vi "ryangosling.vi"(11 "CHASSIS":T6 {"vOmega" format="%10.3f"; "vY" format="%10.3f"; "vX" format="%10.3f"}) -> (1 "out WheelStates":T1[](array[typedef]) {"Angle"."SIN" format="%13.4f"; "Angle"."COS" format="%13.4f"; "Angle"."VALUE" format="%13.4f"}, 3 "out SWERVE_DRIVE_KINEMATICS":T3 {"SavedModuleStates"."Angle"."SIN" format="%13.4f"; "SavedModuleStates"."Angle"."COS" format="%13.4f"; "SavedModuleStates"."Angle"."VALUE" format="%13.4f"; "PrevCoR"."Y" format="%14.3f"; "PrevCoR"."X" format="%14.3f"; "Modules"."Y" format="%14.3f"; "Modules"."X" format="%14.3f"})   [LabVIEW 2023]
uses:
  <vilib>/Rock Robotics/WPI/ThirdParty/JAS_Junk/TrajLib/TypeDef/CHASSIS_SPEEDS.ctl
  <vilib>/Rock Robotics/WPI/ThirdParty/JAS_Junk/TrajLib/TypeDef/SWERVE_DRIVE_KINEMATICS.ctl
  <vilib>/Analysis/Matrix/Datatypes/RealMatrix.ctl
  <vilib>/Rock Robotics/WPI/ThirdParty/JAS_Junk/TrajLib/TypeDef/TRANSLATION2D.ctl
  <vilib>/Rock Robotics/WPI/ThirdParty/JAS_Junk/TrajLib/TypeDef/SWERVE_DRIVE_MODULE_STATE.ctl
  <vilib>/Rock Robotics/WPI/ThirdParty/JAS_Junk/TrajLib/TypeDef/ROTATION2D.ctl
  <vilib>/Rock Robotics/WPI/ThirdParty/JAS_Junk/TrajLib/Rotation2d_Minus.vi
  <vilib>/Rock Robotics/WPI/ThirdParty/JAS_Junk/TrajLib/Rotation2d_GetRadians.vi
  <vilib>/Rock Robotics/WPI/ThirdParty/JAS_Junk/TrajLib/SwerveModuleState_New.vi
  <vilib>/Rock Robotics/WPI/ThirdParty/JAS_Junk/TrajLib/Rotation2d_RotateBy.vi
  <vilib>/Rock Robotics/WPI/ThirdParty/JAS_Junk/TrajLib/Rotation2d_UnaryMinus.vi
  <vilib>/Rock Robotics/WPI/ThirdParty/JAS_Junk/TrajLib/Rotation2d_CreateXY.vi
  <vilib>/Rock Robotics/WPI/ThirdParty/JAS_Junk/TrajLib/Util_CalcDist.vi
  <vilib>/Rock Robotics/WPI/ThirdParty/JAS_Junk/TrajLib/Trajectory_Library.lvlib
  <vilib>/Rock Robotics/WPI/ThirdParty/REV Robotics/REVLib/Typedef/Spark MAX Control Type.ctl
  <vilib>/Analysis/Matrix/NI_Matrix.lvlib
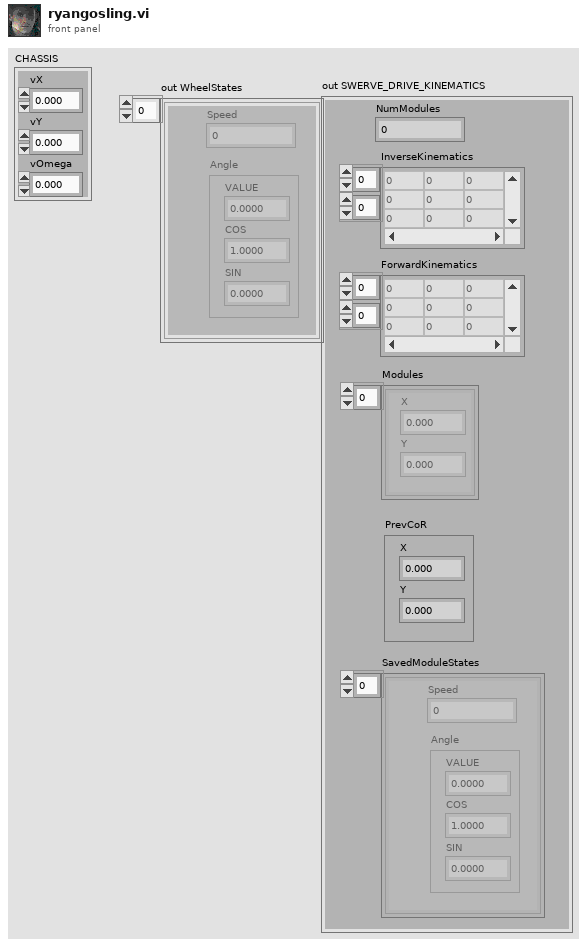
[diagram p1: front panel]
types:
  T1 = typedef "Trajectory_Library.lvlib/SWERVE_DRIVE_MODULE_STATE.ctl" = cluster{"Speed":dbl, "Angle":T2}
  T2 = typedef "Trajectory_Library.lvlib/ROTATION2D.ctl" = cluster{"VALUE":dbl, "COS":dbl, "SIN":dbl}
  T3 = typedef "Trajectory_Library.lvlib/SWERVE_DRIVE_KINEMATICS.ctl" = cluster{"NumModules":i32, "InverseKinematics":T4, "ForwardKinematics":T4, "Modules":T5[], "PrevCoR":T5, "SavedModuleStates":T1[]}
  T4 = typedef "NI_Matrix.lvlib/RealMatrix.ctl" = dbl[][]
  T5 = typedef "Trajectory_Library.lvlib/TRANSLATION2D.ctl" = cluster{"X":dbl, "Y":dbl}
  T6 = typedef "Trajectory_Library.lvlib/CHASSIS_SPEEDS.ctl" = cluster{"vX":dbl, "vY":dbl, "vOmega":dbl}
  T7 = typedef "WPI_MotorControlDeviceRef.ctl" = cluster{"DeviceStatus":errorcluster, "Type":T8, "PWM":cluster{"PWM Channel":T9, "DeadBand":T10}, "CAN":cluster{"Device Number":u8, "SetOutput VI Ref":variant, "GetOutput VI Ref":variant, "Enable VI Ref":variant, "Disable VI Ref":variant, "Data":variant}, "Invert":bool, "DIO PWM":cluster{"PWM \"Enable\" Channel":T9, "DIOChannel":T11, "PWM Rate":dbl}}
  T8 = typedef "WPI_MotorControlType.ctl" = enum16{"PWM", "CAN", "DIO PWM"}
  T9 = typedef "FPGA_DIOPWMChannel.ctl" = enum8{"PWM 0", "PWM 1", "PWM 2", "PWM 3", "PWM 4", "PWM 5", "PWM 6", "PWM 7", "PWM 8", "PWM 9", "PWM MXP 0", "PWM MXP 1", "PWM MXP 2", "PWM MXP 3", "PWM MXP 4", "PWM MXP 5", "PWM MXP 6", "PWM MXP 7", "PWM MXP 8", "PWM MXP 9", "Invalid"}
  T10 = typedef "WPI_PWMDeadband.ctl" = cluster{"Name":string, "maxPositivePwm":i32, "minPositivePwm":i32, "centerPwm":i32, "maxNegativePwm":i32, "minNegativePwm":i32, "angularRange":u16}
  T11 = typedef "FPGA_DIOChannel.ctl" = enum8{"DIO 0", "DIO 1", "DIO 2", "DIO 3", "DIO 4", "DIO 5", "DIO 6", "DIO 7", "DIO 8", "DIO 9", "DIO MXP 0", "DIO MXP 1", "DIO MXP 2", "DIO MXP 3", "DIO MXP 4", "DIO MXP 5", "DIO MXP 6", "DIO MXP 7", "DIO MXP 8", "DIO MXP 9", "DIO MXP 10", "DIO MXP 11", "DIO MXP 12", "DIO MXP 13", "DIO MXP 14", "DIO MXP 15", "SPI Port CS1", "SPI Port CS2", "SPI Port CS3", "SPI Port MISO", "SPI Port MOSI", "Invalid"}
  T12 = typedef "Spark MAX Control Type.ctl" = enum16{"Percent VBus", "Voltage", "Velocity", "Position", "Smart Motion", "Current", "Smart Velocity"}
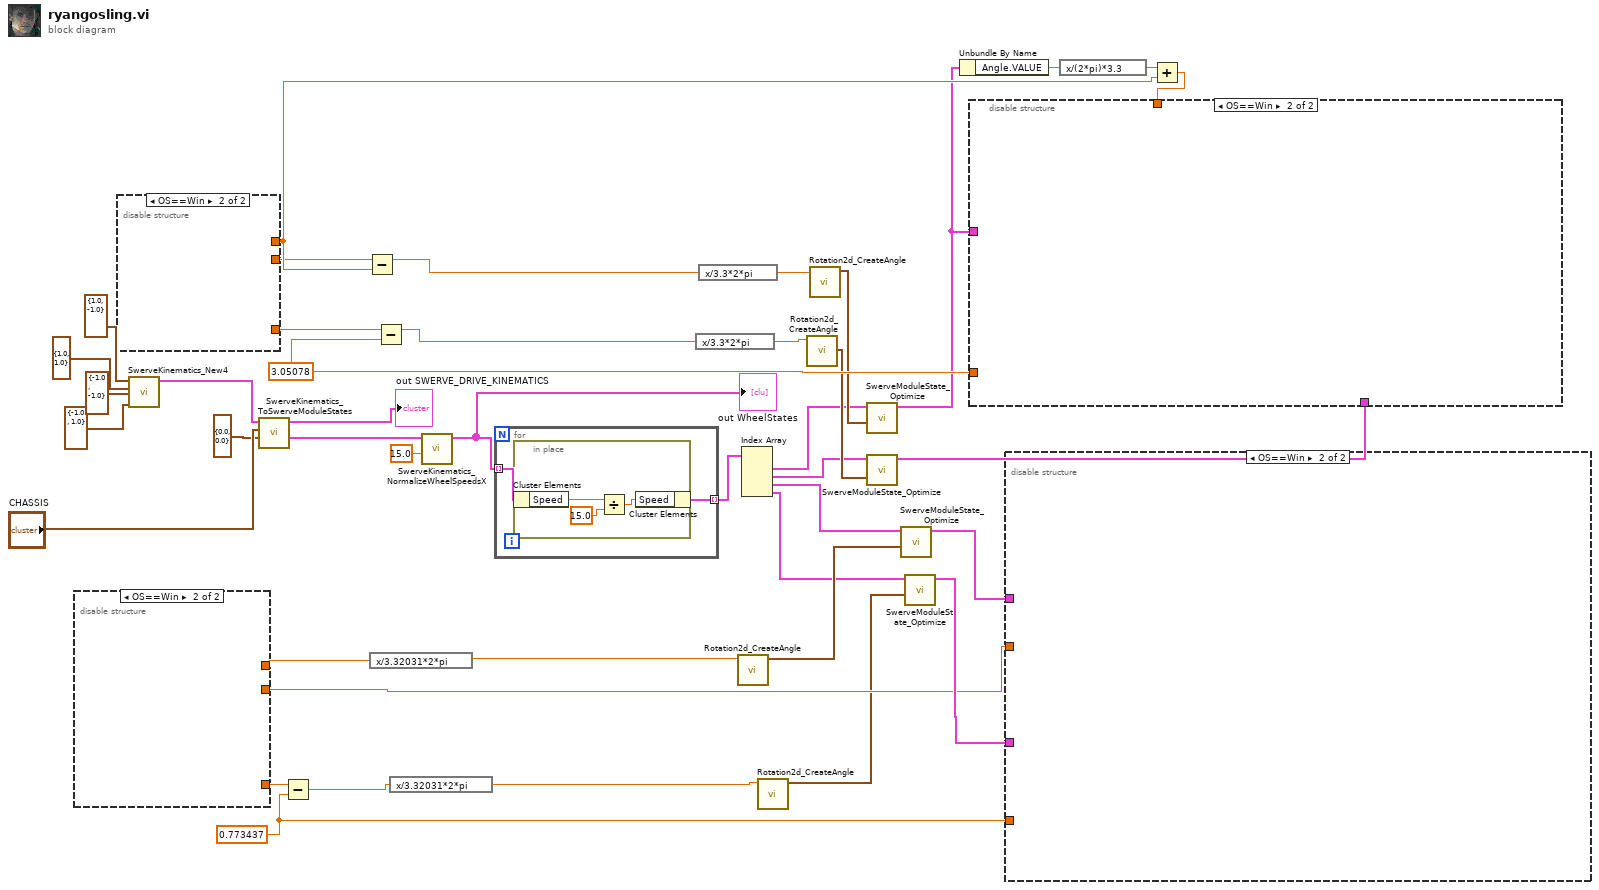
[diagram p0: block diagram]
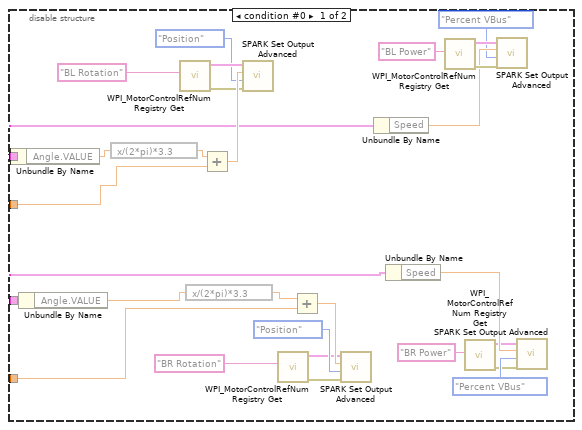
[diagram p2: hidden frame]
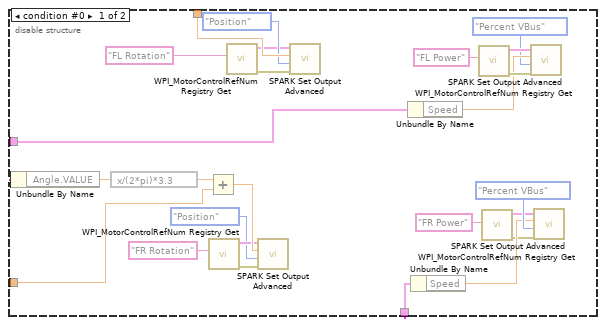
[diagram p3: hidden frame]
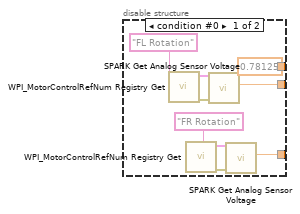
[diagram p4: hidden frame]
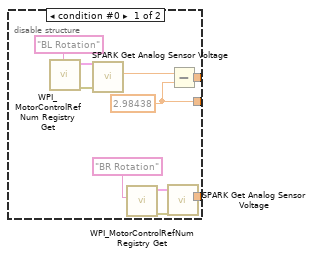
[diagram p5: hidden frame]
diagram:
  w34 = 0.773437 ("x")
  w36 = 3.05078 ("y")
  n1 = disable-structure shown="OS==Win" {
    disable-tunnel: [w52 _] -> w35
    disable-tunnel: [w51 _] -> w32
    disable-tunnel: [w49 _] -> w23
    frame condition #0 {
      w52 = 2.98438 ("y")
      n2 = call <vilib>:"WPI_MotorControlRefNum Registry Get.vi"("refnum name"="BL Rotation") -> ("error out"=w44:errorcluster, "MotorControlDevRef"=w45:T7)  [unwired: 9 in]
      n3 = call <vilib>:"SPARK Get Analog Sensor Voltage.vi"("error in (no error)"=w44, "MotorControlDevRef in"=w45) -> ("Analog Sensor Voltage"=w50:dbl)  [unwired: 6 in, 3 out]
      n4 = call <vilib>:"WPI_MotorControlRefNum Registry Get.vi"("refnum name"="BR Rotation") -> ("error out"=w47:errorcluster, "MotorControlDevRef"=w46:T7)  [unwired: 9 in]
      n5 = call <vilib>:"SPARK Get Analog Sensor Voltage.vi"("error in (no error)"=w47, "MotorControlDevRef in"=w46) -> ("Analog Sensor Voltage"=w49:dbl)  [unwired: 6 in, 3 out]
      n6 = Subtract(x=w50, y=w52) -> (x-y=w51:dbl)
    }
    frame condition #1 (active) {
    }
  }
  n7 = disable-structure shown="OS==Win" {
    disable-tunnel: [0.78125 ("y") _] -> w37
    disable-tunnel: [w60 _] -> w20
    disable-tunnel: [w59 _] -> w17
    frame condition #0 {
      n8 = call <vilib>:"WPI_MotorControlRefNum Registry Get.vi"("refnum name"="FL Rotation") -> ("error out"=w54:errorcluster, "MotorControlDevRef"=w55:T7)  [unwired: 9 in]
      n9 = call <vilib>:"WPI_MotorControlRefNum Registry Get.vi"("refnum name"="FR Rotation") -> ("error out"=w57:errorcluster, "MotorControlDevRef"=w56:T7)  [unwired: 9 in]
      n10 = call <vilib>:"SPARK Get Analog Sensor Voltage.vi"("error in (no error)"=w54, "MotorControlDevRef in"=w55) -> ("Analog Sensor Voltage"=w59:dbl)  [unwired: 6 in, 3 out]
      n11 = call <vilib>:"SPARK Get Analog Sensor Voltage.vi"("error in (no error)"=w57, "MotorControlDevRef in"=w56) -> ("Analog Sensor Voltage"=w60:dbl)  [unwired: 6 in, 3 out]
    }
    frame condition #1 (active) {
    }
  }
  n12 = call <vilib>:"SwerveKinematics_New4.vi"("wheel 3"=T5 {"X"=-1.0, "Y"=1.0} ("wheel 0"), "wheel 2"=T5 {"X"=-1.0, "Y"=-1.0} ("wheel 0"), "wheel 1"=T5 {"X"=1.0, "Y"=1.0} ("wheel 0"), "wheel 0"=T5 {"X"=1.0, "Y"=-1.0}) -> ("SWERVE_DRIVE_KINEMATICS"=w10:T3)  [unwired: 7 in]
  n13 = call <vilib>:"SwerveKinematics_ToSwerveModuleStates.vi"("CenterOfRotation"=T5 {"X"=0.0, "Y"=0.0}, "ChassisSpeeds"="CHASSIS", "in SWERVE_DRIVE_KINEMATICS"=w10) -> ("ModuleStates"=w3:T1[], "out SWERVE_DRIVE_KINEMATICS"=→"out SWERVE_DRIVE_KINEMATICS":T3)  [unwired: 7 in]
  n14 = Subtract(x=w23, y=w34) -> (x-y=w33:dbl)
  n15 = Subtract(x=w17, y=w37) -> (x-y=w31:dbl)
  n16 = expression code="x/3.32031*2*pi"(w32) -> (w25:dbl)
  n17 = Subtract(x=w20, y=w36) -> (x-y=w30:dbl)
  n18 = expression code="x/3.32031*2*pi"(w33) -> (w24:dbl)
  n19 = call <vilib>:"SwerveKinematics_NormalizeWheelSpeedsX.vi"("AttainableMaxSpeed"=15.0, "in WheelStates"=w3) -> ("out WheelStates"=w1:T1[])  [unwired: 9 in]
  "out WheelStates" <- w1
  n20 = for {
    tunnel: w1 -> [w63] mode=indexing
    tunnel: [w62] -> w2 mode=indexing
    n21 = in-place {
      n22 = in-place-cluster #1(w63) -> ("Speed"=w65:dbl)
      n23 = Divide(x=w65, y=15.0) -> (x/y=w66:dbl)
      n24 = in-place-cluster #1("Speed"=w66) -> (w62:T1)
    }
  }
  n25 = expression code="x/3.3*2*pi"(w30) -> (w21:dbl)
  n26 = expression code="x/3.3*2*pi"(w31) -> (w18:dbl)
  n27 = call <vilib>:"Rotation2d_CreateAngle.vi"("Angle"=w25) -> ("ROTATION"=w26:T2)  [unwired: 10 in]
  n28 = Index Array(array=w2) -> (element #1=w13:T1, element #2=w16:T1, element #3=w15:T1, element #4=w14:T1)  [unwired: 4 in]
  n29 = call <vilib>:"Rotation2d_CreateAngle.vi"("Angle"=w24) -> ("ROTATION"=w27:T2)  [unwired: 10 in]
  n30 = call <vilib>:"Rotation2d_CreateAngle.vi"("Angle"=w21) -> ("ROTATION"=w22:T2)  [unwired: 10 in]
  n31 = call <vilib>:"Rotation2d_CreateAngle.vi"("Angle"=w18) -> ("ROTATION"=w19:T2)  [unwired: 10 in]
  n32 = call <vilib>:"SwerveModuleState_Optimize.vi"("CurrentAngle"=w19, "Desired State"=w13) -> ("out SWERVE_DRIVE_MODULE_STATE"=w28:T1)  [unwired: 9 in]
  n33 = call <vilib>:"SwerveModuleState_Optimize.vi"("CurrentAngle"=w22, "Desired State"=w16) -> ("out SWERVE_DRIVE_MODULE_STATE"=w29:T1)  [unwired: 9 in]
  n34 = call <vilib>:"SwerveModuleState_Optimize.vi"("CurrentAngle"=w26, "Desired State"=w15) -> ("out SWERVE_DRIVE_MODULE_STATE"=w38:T1)  [unwired: 9 in]
  n35 = call <vilib>:"SwerveModuleState_Optimize.vi"("CurrentAngle"=w27, "Desired State"=w14) -> ("out SWERVE_DRIVE_MODULE_STATE"=w39:T1)  [unwired: 9 in]
  n36 = Unbundle By Name(w28) -> ("Angle.VALUE"=w41:dbl)
  n37 = disable-structure shown="OS==Win" {
    disable-tunnel: w39 -> [w87 _]
    disable-tunnel: w38 -> [w86 _]
    disable-tunnel: w35 -> [w68 _]
    disable-tunnel: w34 -> [w67 _]
    frame condition #0 {
      n38 = Unbundle By Name(w86) -> ("Angle.VALUE"=w89:dbl)
      n39 = Unbundle By Name(w87) -> ("Angle.VALUE"=w94:dbl)
      n40 = expression code="x/(2*pi)*3.3"(w89) -> (w90:dbl)
      n41 = call <vilib>:"WPI_MotorControlRefNum Registry Get.vi"("refnum name"="BL Rotation") -> ("error out"=w75:errorcluster, "MotorControlDevRef"=w74:T7)  [unwired: 9 in]
      n42 = expression code="x/(2*pi)*3.3"(w94) -> (w92:dbl)
      n43 = Add(x=w90, y=w68) -> (x+y=w91:dbl)
      n44 = call <vilib>:"SPARK Set Output Advanced.vi"("error in (no error)"=w75, "Control Mode"=Spark_MAX_Control_Type."Position", "Setpoint"=w91, "MotorControlDevRef"=w74) -> ()  [unwired: 6 in, 2 out]
      n45 = call <vilib>:"WPI_MotorControlRefNum Registry Get.vi"("refnum name"="BR Rotation") -> ("error out"=w70:errorcluster, "MotorControlDevRef"=w71:T7)  [unwired: 9 in]
      n46 = Add(x=w92, y=w67) -> (x+y=w93:dbl)
      n47 = call <vilib>:"SPARK Set Output Advanced.vi"("error in (no error)"=w70, "Control Mode"=Spark_MAX_Control_Type."Position", "Setpoint"=w93, "MotorControlDevRef"=w71) -> ()  [unwired: 6 in, 2 out]
      n48 = Unbundle By Name(w86) -> ("Speed"=w78:dbl)
      n49 = Unbundle By Name(w87) -> ("Speed"=w83:dbl)
      n50 = call <vilib>:"WPI_MotorControlRefNum Registry Get.vi"("refnum name"="BL Power") -> ("error out"=w80:errorcluster, "MotorControlDevRef"=w79:T7)  [unwired: 9 in]
      n51 = call <vilib>:"WPI_MotorControlRefNum Registry Get.vi"("refnum name"="BR Power") -> ("error out"=w81:errorcluster, "MotorControlDevRef"=w82:T7)  [unwired: 9 in]
      n52 = call <vilib>:"SPARK Set Output Advanced.vi"("error in (no error)"=w80, "Control Mode"=Spark_MAX_Control_Type."Percent VBus", "Setpoint"=w78, "MotorControlDevRef"=w79) -> ()  [unwired: 6 in, 2 out]
      n53 = call <vilib>:"SPARK Set Output Advanced.vi"("error in (no error)"=w81, "Control Mode"=Spark_MAX_Control_Type."Percent VBus", "Setpoint"=w83, "MotorControlDevRef"=w82) -> ()  [unwired: 6 in, 2 out]
    }
    frame condition #1 (active) {
    }
  }
  n54 = expression code="x/(2*pi)*3.3"(w41) -> (w40:dbl)
  n55 = Add(x=w40, y=w37) -> (x+y=w42:dbl)
  n56 = disable-structure shown="OS==Win" {
    disable-tunnel: w42 -> [w116 _]
    disable-tunnel: w36 -> [w97 _]
    disable-tunnel: w29 -> [w96 _]
    disable-tunnel: w28 -> [w95 _]
    frame condition #0 {
      n57 = Unbundle By Name(w96) -> ("Angle.VALUE"=w117:dbl)
      n58 = expression code="x/(2*pi)*3.3"(w117) -> (w118:dbl)
      n59 = Add(x=w118, y=w97) -> (x+y=w119:dbl)
      n60 = call <vilib>:"WPI_MotorControlRefNum Registry Get.vi"("refnum name"="FR Rotation") -> ("error out"=w104:errorcluster, "MotorControlDevRef"=w103:T7)  [unwired: 9 in]
      n61 = call <vilib>:"WPI_MotorControlRefNum Registry Get.vi"("refnum name"="FL Rotation") -> ("error out"=w99:errorcluster, "MotorControlDevRef"=w100:T7)  [unwired: 9 in]
      n62 = call <vilib>:"SPARK Set Output Advanced.vi"("error in (no error)"=w104, "Control Mode"=Spark_MAX_Control_Type."Position", "Setpoint"=w119, "MotorControlDevRef"=w103) -> ()  [unwired: 6 in, 2 out]
      n63 = call <vilib>:"SPARK Set Output Advanced.vi"("error in (no error)"=w99, "Control Mode"=Spark_MAX_Control_Type."Position", "Setpoint"=w116, "MotorControlDevRef"=w100) -> ()  [unwired: 6 in, 2 out]
      n64 = Unbundle By Name(w95) -> ("Speed"=w108:dbl)
      n65 = Unbundle By Name(w96) -> ("Speed"=w113:dbl)
      n66 = call <vilib>:"WPI_MotorControlRefNum Registry Get.vi"("refnum name"="FL Power") -> ("error out"=w110:errorcluster, "MotorControlDevRef"=w109:T7)  [unwired: 9 in]
      n67 = call <vilib>:"WPI_MotorControlRefNum Registry Get.vi"("refnum name"="FR Power") -> ("error out"=w111:errorcluster, "MotorControlDevRef"=w112:T7)  [unwired: 9 in]
      n68 = call <vilib>:"SPARK Set Output Advanced.vi"("error in (no error)"=w110, "Control Mode"=Spark_MAX_Control_Type."Percent VBus", "Setpoint"=w108, "MotorControlDevRef"=w109) -> ()  [unwired: 6 in, 2 out]
      n69 = call <vilib>:"SPARK Set Output Advanced.vi"("error in (no error)"=w111, "Control Mode"=Spark_MAX_Control_Type."Percent VBus", "Setpoint"=w113, "MotorControlDevRef"=w112) -> ()  [unwired: 6 in, 2 out]
    }
    frame condition #1 (active) {
    }
  }
